vi "measureDelayBetweenChannels.vi"(7 "Measurement time (s)":dbl=2.0 caption="Delay Time (s)", 8 "error in (no error)":errorcluster, 9 "channel_2":i32=2, 10 "channel_1":i32=1, 11 "TimeTagger ref in":refnum<k24>) -> (0 "error out":errorcluster, 2 "measured delay, ps":i64, 3 "TimeTagger ref out":refnum<k24>)   [LabVIEW 2014]
doc: "This code uses Correlation measurement \nto determine propagation delay between two correlated signals."
uses:
  SwabianInstruments.TimeTagger
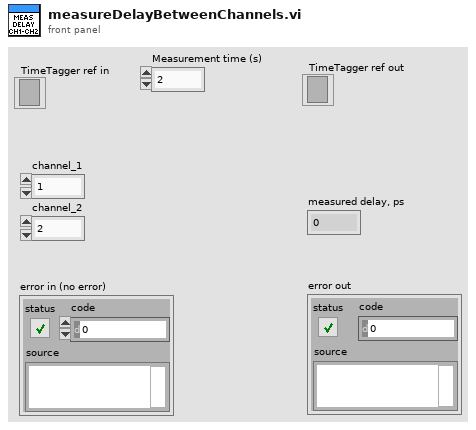
[diagram p1: front panel]
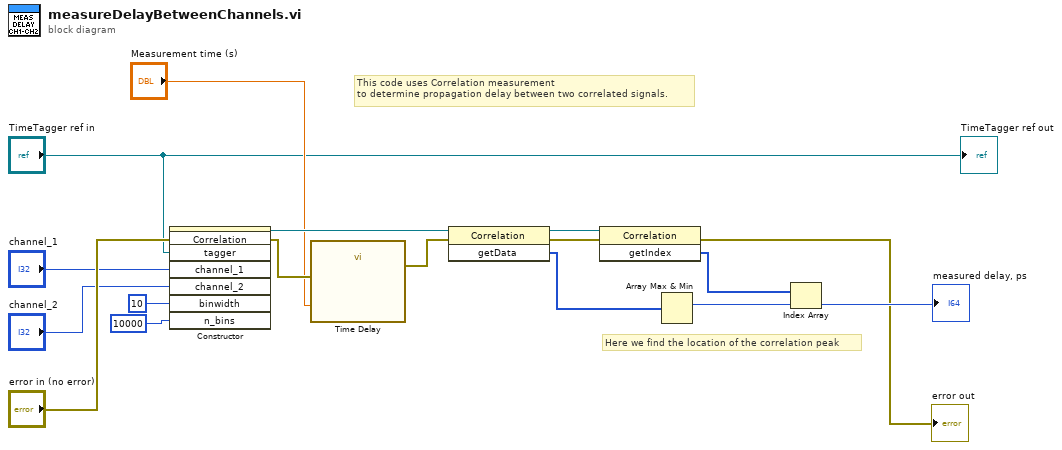
[diagram p0: block diagram]
diagram:
  # "Here we find the location of the correlation peak"
  # "This code uses Correlation measurement \nto determine propagation delay between two correlated signals."
  n1 = constructor class="Correlation"(error in="error in (no error)", "tagger"="TimeTagger ref in", "channel_1"="channel_1", "channel_2"="channel_2", "binwidth"=i64 10, "n_bins"=10000) -> (reference out=w12:refnum<k24>, error out=w11:errorcluster)  [unwired: 2 in, 6 out]
  n2 = call "Time Delay"("error in (no error)"=w11, "Delay Time (s)"="Measurement time (s)") -> ("error out"=w10:errorcluster)  [unwired: 9 in]
  n3 = invoke class="Correlation" method="getData"(reference=w12, error in=w10) -> (reference out=w4:refnum<k24>, error out=w5:errorcluster, "getData"=w13:i32[])  [unwired: 1 in]
  n4 = invoke class="Correlation" method="getIndex"(reference=w4, error in=w5) -> (error out=→"error out":errorcluster, "getIndex"=w15:i64[])  [unwired: 1 in, 1 out]
  n5 = Array Max & Min(array=w13) -> (max index (indices)=w14:i32)  [unwired: 3 out]
  n6 = Index Array(array=w15, index=w14) -> (element=→"measured delay, ps":i64)
  "TimeTagger ref out" <- "TimeTagger ref in"
